vi "Launch Event Reporter.vi"(8 "error in (no error)":errorcluster, 11 "Volatus Core in":refnum<class "Volatus Core.lvclass">) -> (0 "error out":errorcluster, 3 "Volatus Core out":refnum<class "Volatus Core.lvclass">)   [LabVIEW 2020, in "Volatus.lvlib" / "Volatus Core.lvclass"]
uses:
  Volatus Core.lvclass
  C:/dev/lv20CE/relink/lv-volatus/Volatus/Module/Module.lvclass
  VolatusConfig/VolatusConfigElement/VolatusConfigElement.lvclass
  Module/Module.lvclass/Module.ctl
  VolatusConfig/VolatusConfigElement/VolatusConfigElement.lvclass/VolatusConfigElement.ctl
  VolatusAPI/VolatusAPI.lvclass/VolatusAPI.ctl
  Volatus Core.lvclass/Volatus Core.ctl
  VolatusConfig/VolatusConfigElement/Element.vi
  MessageQ/MessageQ.lvclass
  C:/dev/lv20CE/relink/lv-volatus/Volatus/Volatus Core/Volatus Core.lvclass
  Module/Module.lvclass
  VolatusAPI/VolatusAPI.lvclass
  VectoEventBridge/VectoEventBridge.lvclass
  Event Reporter Module/Event Reporter Module.lvclass
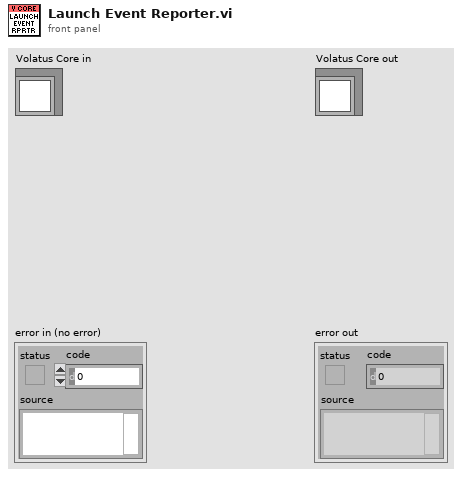
[diagram p1: front panel]
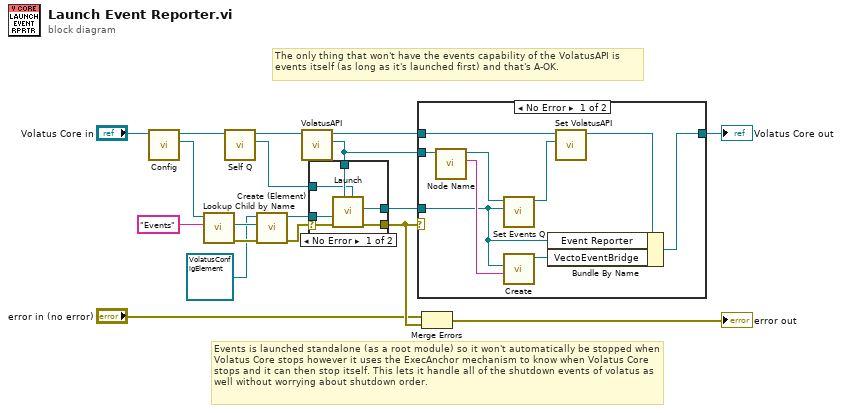
[diagram p0: block diagram]
diagram:
  # "Events is launched standalone (as a root module) so it won't automatically be stopped when Volatus Core stops however it uses the ExecAnchor mechanism to know when Volatus Core stops and it can then stop itself. This lets it handle all of the shutdown events of volatus as well without worrying about shutdown order."
  # "The only thing that won't have the events capability of the VolatusAPI is events itself (as long as it's launched first) and that's A-OK."
  n1 = call "Config.vi"("Module in"="Volatus Core in") -> ("Config"=w17:refnum<class "VolatusConfigElement.lvclass">, "Module out"=w5:refnum<class "Volatus Core.lvclass">)  [unwired: 9 in]
  n2 = call "Lookup Child by Name.vi"("Child Name"="Events" ("Name"), "VolatusConfigElement in"=w17) -> ("error out"=w10:errorcluster, "Child"=w9:refnum<class "Config Element.lvclass">)  [unwired: 6 in, 2 out]
  n3 = call "Self Q.vi"("Module in"=w5) -> ("Self Q"=w1:refnum<class "MessageQ.lvclass">, "Module out"=w2:refnum<class "Volatus Core.lvclass">)  [unwired: 9 in]
  n4 = call "Create (Element).vi"("error in (no error)"=w10, "Element"=w9, "VolatusConfigElement in"=refnum<class "VolatusConfigElement.lvclass"> refnum) -> ("error out"=w8:errorcluster, "VolatusConfigElement out"=w7:refnum<class "VolatusConfigElement.lvclass">)  [unwired: 7 in]
  n5 = call "VolatusAPI.vi"("Module in"=w2) -> ("VolatusAPI"=w3:refnum<class "VolatusAPI.lvclass">, "Module out"=w4:refnum<class "Volatus Core.lvclass">)  [unwired: 9 in]
  n6 = case shown="No Error" w8 {
    selector: w8 -> [w22 w25]
    tunnel: w7 -> [w21 _]
    tunnel: [w23 _] -> w15
    tunnel: [w24 w25] -> w13
    tunnel: w3 -> [w20 _]
    tunnel: w1 -> [w19 _]
    frame No Error {
      n7 = call "Launch.vi"("Status Q"=w19, "VolatusAPI"=w20, "error in (no error)"=w22, "Config"=w21) -> ("error out"=w24:errorcluster, "MessageQ"=w23:refnum<class "MessageQ.lvclass">)  [unwired: 6 in]
    }
    frame Error {
    }
  }
  n8 = case shown="No Error" w13 {
    tunnel: w15 -> [w26 _]
    tunnel: w4 -> [w34 w35]
    tunnel: [w31 w35] -> w14
    tunnel: w3 -> [w27 _]
    frame No Error {
      n9 = call "Node Name.vi"("VolatusAPI in"=w27) -> ("Node Name"=w28:string, "VolatusAPI out"=w29:refnum<class "VolatusAPI.lvclass">)  [unwired: 8 in, 1 out]
      n10 = call "Set Events Q.vi"("Events Q"=w26, "VolatusAPI in"=w29) -> ("VolatusAPI out"=w33:refnum<class "VolatusAPI.lvclass">)  [unwired: 9 in]
      n11 = call "Create.vi"("Node"=w28, "MsgQ"=w26) -> ("VectoEventBridge out"=w30:refnum<class "VectoEventBridge.lvclass">)  [unwired: 8 in, 1 out]
      n12 = call "Set VolatusAPI.vi"("VolatusAPI"=w33, "Module in"=w34) -> ("Module out"=w32:refnum<class "Volatus Core.lvclass">)  [unwired: 9 in]
      n13 = Bundle By Name(cluster=w32, "Event Reporter"=w26, "VectoEventBridge"=w30) -> (w31:refnum<class "Volatus Core.lvclass">)
    }
    frame Error {
    }
  }
  "Volatus Core out" <- w14
  n14 = Merge Errors("error in (no error)", w13) -> (→"error out":errorcluster)
